vi "generate channels from UI.vi"(8 "error in":errorcluster, 11 "VI Refnum":refnum<vi>) -> (0 "error out":errorcluster, 2 "channels":refnum<class "TBM channel.lvclass">[](array[class]))   [LabVIEW 2015, in "UI Reference configuration.lvclass"]
uses:
  UI Reference configuration.lvclass
  <vilib>/NI/Tag Bus Module Framework/channel/TBM channel.lvclass
  <vilib>/NI/Tag Bus Module Framework/channel/channel classification.ctl
  <vilib>/NI/Tag Bus/tag/Data Type.ctl
  <vilib>/Utility/VariantDataType/VariantType.lvlib
  <vilib>/NI/Tag Bus/tag/tag descriptor.lvclass
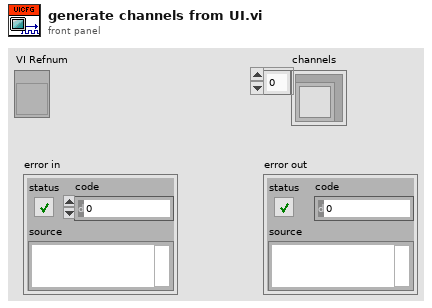
[diagram p1: front panel]
types:
  T1 = typedef "TBM channel.lvclass/channel classification.ctl" = enum16{"input data", "output data", "processing parameter", "processing result"}
  T2 = typedef "tag bus.lvlib/tag descriptor.lvclass/Data Type.ctl" = enum16{"Double", "Single", "I64", "I32", "I16", "I8", "U64", "U32", "U16", "U8", "Boolean", "String", "Array of Double", "Array of Single", "Array of I64", "Array of I32", "Array of I16", "Array of I8", "Array of U64", "Array of U32", "Array of U16", "Array of U8", "Array of Boolean", "Array of String"}
  T3 = typedef "VariantType.lvlib/Type.ctl" = enum8{"Invalid Type", "Void", "I8", "I16", "I32", "I64", "U8", "U16", "U32", "U64", "Single Float", "Double Float", "Extended Float", "Single Complex", "Double Complex", "Extended Complex", "Enum U8", "Enum U16", "Enum U32", "Enum U64", "Single Float With Unit", "Double Float With Unit", "Extended Float With Unit", "Single Complex with Unit", "Double Complex with Unit", "Extended Complex with Unit", "Boolean", "String", "Path", "Picture", "Tag", "Array", "Cluster", "Variant", "LV Variant", "Waveform", "Timestamp", "Digital Waveform", "Digital Data", "ExpressData", "Refnum", "External Data", "VI", "Poly VI", "LabVIEW Class Instance", "Fixed Point"}
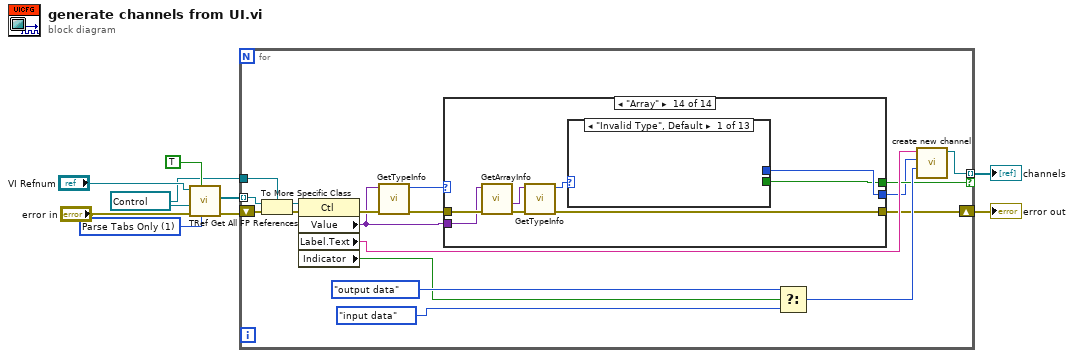
[diagram p0: block diagram]
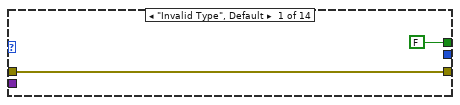
[diagram p2: hidden frame]
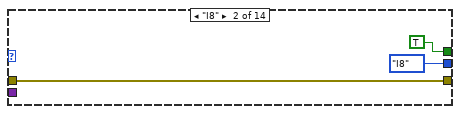
[diagram p3: hidden frame]
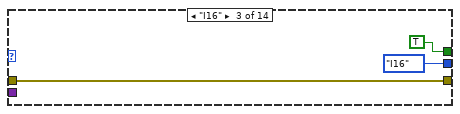
[diagram p4: hidden frame]
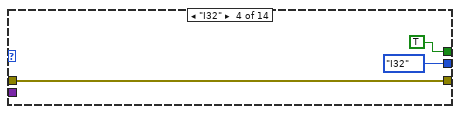
[diagram p5: hidden frame]
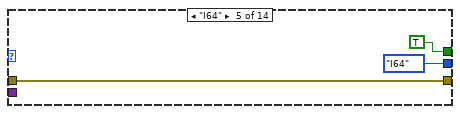
[diagram p6: hidden frame]
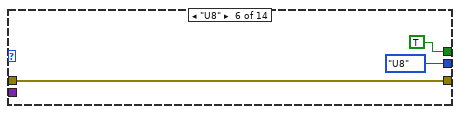
[diagram p7: hidden frame]
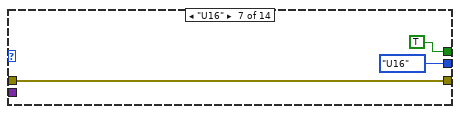
[diagram p8: hidden frame]
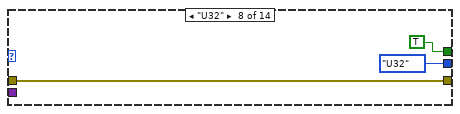
[diagram p9: hidden frame]
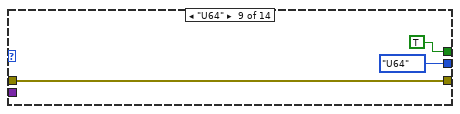
[diagram p10: hidden frame]
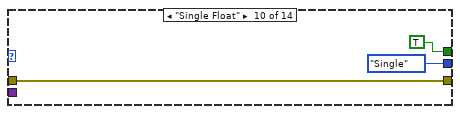
[diagram p11: hidden frame]
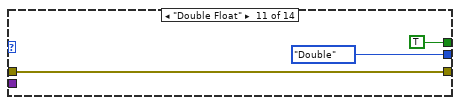
[diagram p12: hidden frame]
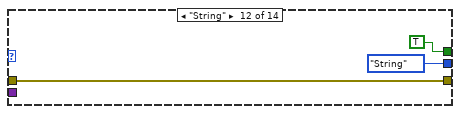
[diagram p13: hidden frame]
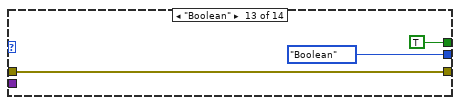
[diagram p14: hidden frame]
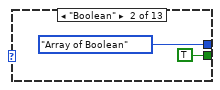
[diagram p15: hidden frame]
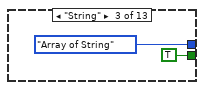
[diagram p16: hidden frame]
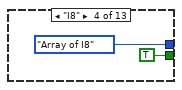
[diagram p17: hidden frame]
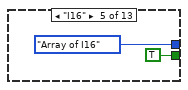
[diagram p18: hidden frame]
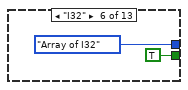
[diagram p19: hidden frame]
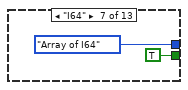
[diagram p20: hidden frame]
diagram:
  w6 = u16 1 items=["Parse All", "Parse Tabs Only"] ("Parsing Rule")
  w3 = refnum<vi> refnum ("Ctl Refnum")
  n1 = call <vilib>:"TRef Get All FP References.vi"("Parsing Rule"=w6, "Ignore Decorations?"=TRUE, "error in (no error)"="error in", "GObj Refnum"=w3, "VI Refnum"="VI Refnum") -> ("error out"=w2:errorcluster, "All FP Objects"=w1:refnum<vi>[])  [unwired: 2 in, 3 out]
  n2 = for {
    shift-right: [w15] -> w9
    shift-left: w2 -> [w14]
    tunnel: [w27] -> w8 mode=indexing if=w17
    tunnel: w3 -> [w12]
    tunnel: w1 -> [w10] mode=indexing
    n3 = To More Specific Class(target class=w12, reference=w10, error in=w14) -> (specific class reference=w11:refnum<vi>, error out=w13:errorcluster)
    n4 = property class="Ctl"(reference=w11, error in=w13) -> (error out=w21:errorcluster, "Value"=w18:variant, "Label.Text"=w26:string, "Indicator"=w23:bool)  [unwired: 1 out]
    n5 = call <vilib>:"GetTypeInfo.vi"("error in (no error)"=w21, "Variant"=w18) -> ("error out"=w19:errorcluster, "Type Enum"=w20:T3)  [unwired: 5 in, 3 out]
    n6 = case shown="\"Array\"" w20 {
      tunnel: w19 -> [w28 w30 w33 w36 w39 w42 w45 w48 w51 w54 w57 w60 w63 w73]
      tunnel: w18 -> [_ _ _ _ _ _ _ _ _ _ _ _ _ w72]
      tunnel: [FALSE TRUE TRUE TRUE TRUE TRUE TRUE TRUE TRUE TRUE TRUE TRUE TRUE w66] -> w17
      tunnel: [_ Data_Type."I8" ("data type") Data_Type."I16" ("data type") Data_Type."I32" ("data type") Data_Type."I64" ("data type") Data_Type."U8" ("data type") Data_Type."U16" ("data type") Data_Type."U32" ("data type") Data_Type."U64" ("data type") Data_Type."Single" ("data type") Data_Type."Double" ("data type") Data_Type."String" ("data type") Data_Type."Boolean" ("data type") w67] -> w16
      tunnel: [w28 w30 w33 w36 w39 w42 w45 w48 w51 w54 w57 w60 w63 w69] -> w15
      frame "Invalid Type", Default {
      }
      frame "I8" {
      }
      frame "I16" {
      }
      frame "I32" {
      }
      frame "I64" {
      }
      frame "U8" {
      }
      frame "U16" {
      }
      frame "U32" {
      }
      frame "U64" {
      }
      frame "Single Float" {
      }
      frame "Double Float" {
      }
      frame "String" {
      }
      frame "Boolean" {
      }
      frame "Array" {
        n7 = call <vilib>:"GetArrayInfo.vi"("error in (no error)"=w73, "Variant"=w72) -> ("error out"=w71:errorcluster, "ArrayElement"=w70:variant)  [unwired: 6 in, 2 out]
        n8 = call <vilib>:"GetTypeInfo.vi"("error in (no error)"=w71, "Variant"=w70) -> ("error out"=w69:errorcluster, "Type Enum"=w68:T3)  [unwired: 5 in, 3 out]
        n9 = case shown="\"Invalid Type\", Default" w68 {
          tunnel: [_ Data_Type."Array of Boolean" ("data type") Data_Type."Array of String" ("data type") Data_Type."Array of I8" ("data type") Data_Type."Array of I16" ("data type") Data_Type."Array of I32" ("data type") Data_Type."Array of I64" ("data type") Data_Type."Array of U8" ("data type") Data_Type."Array of U16" ("data type") Data_Type."Array of U32" ("data type") Data_Type."Array of U64" ("data type") Data_Type."Array of Single" ("data type") Data_Type."Array of Double" ("data type")] -> w67
          tunnel: [_ TRUE TRUE TRUE TRUE TRUE TRUE TRUE TRUE TRUE TRUE TRUE TRUE] -> w66
          frame "Invalid Type", Default {
          }
          frame "Boolean" {
          }
          frame "String" {
          }
          frame "I8" {
          }
          frame "I16" {
          }
          frame "I32" {
          }
          frame "I64" {
          }
          frame "U8" {
          }
          frame "U16" {
          }
          frame "U32" {
          }
          frame "U64" {
          }
          frame "Single Float" {
          }
          frame "Double Float" {
          }
        }
      }
    }
    n10 = Select(t=channel_classification."output data" ("channel classification"), s=w23, f=channel_classification."input data" ("channel classification")) -> (s? t:f=w22:T1)
    n11 = call <vilib>:"create new channel.vi"("channel classification"=w22, "data type"=w16, "channel name"=w26) -> ("channel"=w27:refnum<class "TBM channel.lvclass">)  [unwired: 8 in]
  }
  "error out" <- w9
  "channels" <- w8
